vi "Send Plugin Error.vi"(8 "error in (no error)":errorcluster, 9 "timeout in ms (0)":i32 format="%d ms", 10 "error":errorcluster, 11 "Plugin Interface in":refnum<class "Plugin Interface.lvclass">) -> (0 "error out":errorcluster, 3 "Plugin Interface out":refnum<class "Plugin Interface.lvclass">)   [LabVIEW 2017, in "DSF Core.lvlib" / "Plugin Interface.lvclass"]
uses:
  Plugin Interface.lvclass
  C:/Git/DSF/Data Sharing Framework Core/Classes/Interfaces/Interface/Interface.lvclass
  Interface/Interface.lvclass/Interface.ctl
  Interface/Write Error Queue.vi
  Dispatcher/Error Timeout.vi
  Interface/Interface.lvclass
  DSF Core.lvlib
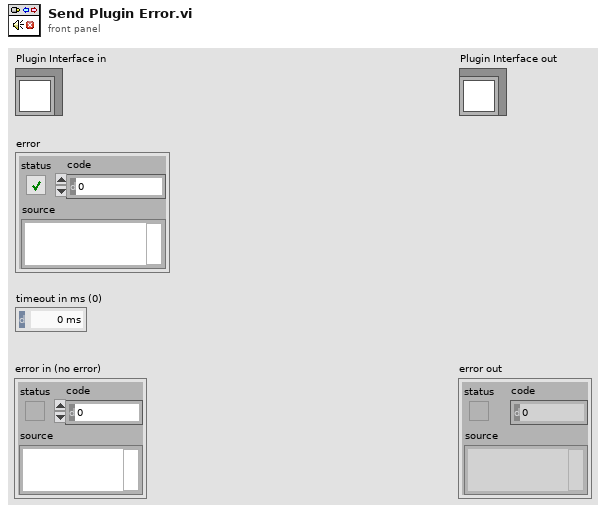
[diagram p1: front panel]
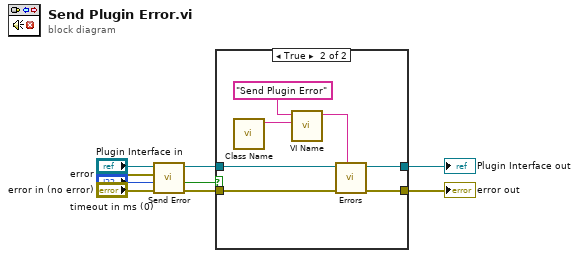
[diagram p0: block diagram]
diagram:
  n1 = call "Send Error.vi"("error in (no error)"="error in (no error)", "timeout in ms (0)"="timeout in ms (0)", "error"="error", "Interface in"="Plugin Interface in") -> ("error out"=w4:errorcluster, "timed out?"=w1:bool, "Interface out"=w5:refnum<class "Plugin Interface.lvclass">)  [unwired: 5 in]
  n2 = case shown="True" w1 {
    tunnel: w4 -> [w10 w17]
    tunnel: w5 -> [w11 w18]
    tunnel: [w11 w16] -> w3
    tunnel: [w10 w15] -> w2
    frame False {
    }
    frame True {
      n3 = call "Class Name.vi"() -> ("class name"=w14:string)  [unwired: 11 in]
      n4 = call "VI Name.vi"("class name (\"\")"=w14, "vi name"="Send Plugin Error" ("error source vi name")) -> ("full VI name"=w12:string)  [unwired: 9 in]
      n5 = call-poly "Errors.vi"("error source vi name"=w12, "error in (no error)"=w17, "Interface in"=w18) -> ("error out"=w15:errorcluster, "Interface out"=w16:refnum<class "Plugin Interface.lvclass">)  [unwired: 7 in]
    }
  }
  "error out" <- w2
  "Plugin Interface out" <- w3
